vi "QAM_1.vi"() -> ()   [LabVIEW 2019]
uses:
  <vilib>/addons/Modulation/Analog/support/mod_Set Error Source.vi
  <vilib>/addons/Modulation/Digital/Support/Common/Validators/mod_AWGN Validate.vi
  <vilib>/addons/Modulation/Digital/Impairments/subVIs/mod_createSeeds.vi
  <vilib>/addons/Modulation/Digital/Support/Common/Validators/mod_Validate Samples Per Symbol.vi
  <vilib>/addons/Modulation/Analog/support/Validators/mod_Validate Complex Waveform.vi
  <vilib>/addons/Modulation/Analog/support/Validators/mod_WFErrorHandler.vi
  <vilib>/addons/Modulation/Digital/General/MT Generate QAM System Parameters(M).vi
  <vilib>/addons/Modulation/Digital/Support/Common/Validators/mod_Generate Filter Coefficients Validate.vi
  <vilib>/addons/Modulation/Digital/General/subVIs/mod_Generate Filter Coefficients.vi
  <vilib>/addons/Modulation/Digital/General/subVIs/mod_Generate Bits PN Sequence.vi
  <vilib>/Analysis/1siggen.llb/Gaussian White Noise (obs 90).vi
  <vilib>/addons/Modulation/Analog/MT Upconvert Baseband (Real).vi
  <vilib>/express/express analysis/Spectral/Block/exnSpectralBlock spectral measurements RMS poly.vi
  <vilib>/express/express analysis/Spectral/Block/exnSpectralBlock spectral measurements RMS DDT.vi
  <vilib>/express/express analysis/Spectral/XNode/ExpressSpectralMeasurementsBlockNode.xnode
  <vilib>/addons/Modulation/niDMT.lvlib
  <vilib>/addons/Modulation/niAMT.lvlib
panel:
  in  "pulse shaping filter (none)":T1(ring)
  in  "?":T2(tab)
  out "Upconverted Waveform":waveform(dbl)(graph)
  out "Constellation Graph":T3(graph)
  out "FFT (RMS)":dynamicdata(graph)
  out "Match Found?":bool
  in  "carrier frequency (Hz)":dbl min=-0.5 max=0.5 format="%.0p"
  in  "stop":bool
  in  "autoscale":bool
  in  "Eb/N0 (10 dB)":dbl=10.0 format="%.0p"
  out "Demodulated String":string
  in  "symbol rate (Hz)":dbl=1.0 format="%.0p"
  in  "Add Bit Padding":bool
  in  "Message to send":string
  in  "M-QAM (16)":u16(ring) items=["4"=4, "8"=8, "16"=16, "32"=32]
  in  "Reset":bool
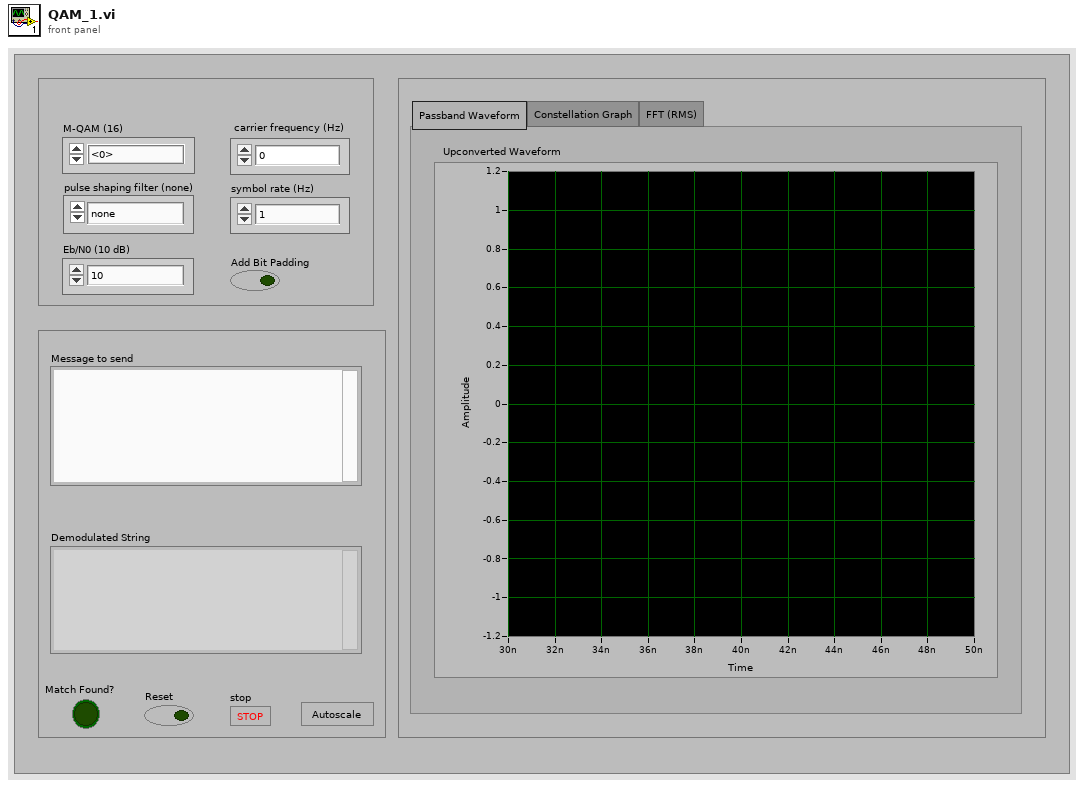
[diagram p1: front panel]
types:
  T1 = enum16{"none", "Raised Cosine", "Root Raised Cos", "Gaussian"}
  T2 = enum32{"Passband Waveform", "Constellation Graph", "FFT (RMS)"}
  T3 = cluster{"Decimated Array":dbl[], "Decimated Array":dbl[]}[]
  T4 = enum16{"FSK", "PSK", "QAM", "MSK", "PAM", "ASK", "CPM"}
  T5 = cluster{"averaging mode":u16, "weighting mode":u16, "number of averages":u32}
  T6 = cluster{"dB On (F)":bool, "unwrap phase (F)":bool, "convert to degree (F)":bool}
  T7 = cluster{"samples per symbol (16)":i32, "symbol map":cdb[]}
  T8 = typedef "niAMT.lvlib/Complex Data Waveform.ctl" = cluster{"t0":dbl, "dt":dbl, "Y":cdb[]}
  T9 = cluster{"constellation":dbl[], "oversampled data":dbl[]}[]
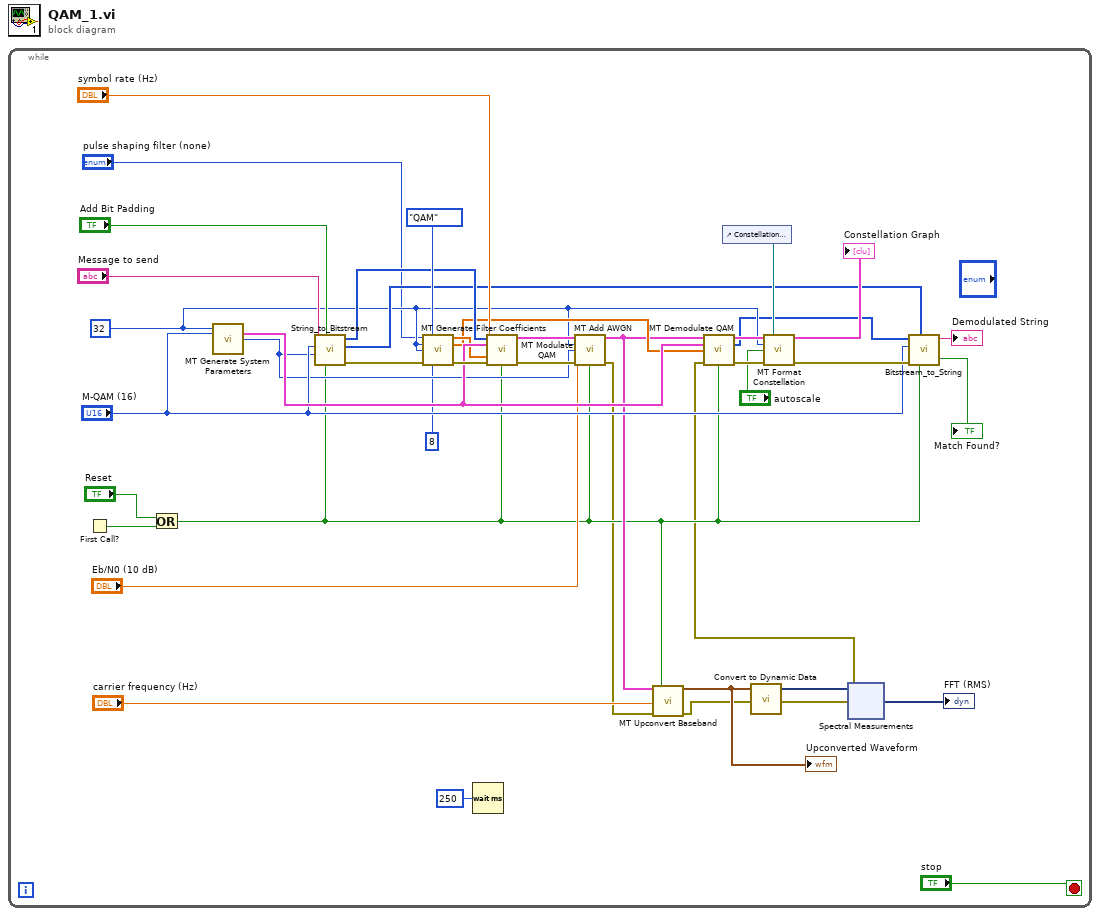
[diagram p0: block diagram]
diagram:
  n1 = while {
    stop <- "stop" stop-if-true
    w13 = 32 ("samples per symbol (16)")
    n2 = First Call?() -> (First Call?: T/F=w38:bool)
    n3 = Or(x="Reset", y=w38) -> (x .or. y?=w5:bool)
    n4 = call-poly <vilib>:"MT Generate System Parameters.vi"("samples per symbol (16)"=w13, "M-QAM (16)"="M-QAM (16)") -> ("QAM system parameters"=w23:T7, "bits per symbol"=w20:i32)  [unwired: 11 in, 1 out]
    n5 = call "String_to_Bitstream.vi"("Reset"=w5, "Add Bit Padding"="Add Bit Padding", "Guard Bits to Add"=w20, "M-ary (16)"="M-QAM (16)", "InputStrig"="Message to send") -> ("error out"=w31:errorcluster, "Character Array"=w32:u8[], "Bitstream (with Guard Bits)"=w33:i8[])  [unwired: 1 in, 2 out]
    n6 = call <vilib>:"MT Generate Filter Coefficients.vi"("pulse shaping filter (none)"="pulse shaping filter (none)", "modulation type"=T4."QAM", "pulse shaping samples per symbol (16)"=w13, "matched samples per symbol (16)"=w13, "error in (no error)"=w31, "filter length (symbols)"=8) -> ("pulse shaping filter coefficients"=w19:dbl[], "matched filter coefficients"=w18:dbl[], "error out"=w30:errorcluster)  [unwired: 7 in]
    n7 = Wait (ms)(milliseconds to wait=u32 250) -> ()  [unwired: 1 out]
    n8 = call <vilib>:"MT Modulate QAM.vi"("input bit stream"=w33, "QAM system parameters"=w23, "symbol rate (Hz)"="symbol rate (Hz)", "pulse shaping filter coefficients"=w19, "error in (no error)"=w30, "reset? (T)"=w5) -> ("output complex waveform"=w24:T8, "error out"=w29:errorcluster)  [unwired: 7 in, 1 out]
    n9 = call <vilib>:"MT Add AWGN.vi"("input complex waveform"=w24, "samples per symbol (16)"=w13, "bits per symbol (1)"=w20, "Eb/N0 (10 dB)"="Eb/N0 (10 dB)", "error in (no error)"=w29, "reset? (T)"=w5) -> ("output complex waveform"=w7:T8, "error out"=w4:errorcluster)  [unwired: 7 in, 1 out]
    n10 = call-poly <vilib>:"MT Upconvert Baseband.vi"("baseband waveform (complex)"=w7, "reset? (F)"=w5, "carrier frequency (Hz)"="carrier frequency (Hz)", "error in (no error)"=w4) -> ("passband waveform"=w16:waveform(dbl), "error out"=w3:errorcluster)  [unwired: 10 in]
    "Upconverted Waveform" <- w16
    n11 = control-ref of="Constellation Graph"() -> (w41:refnum<vi>)
    n12 = call "Convert to Dynamic Data"("Waveform"=w16) -> ("Dynamic Data Type"=w17:dynamicdata)  [unwired: 3 in]
    n13 = xnode "Spectral Measurements"("Signals"=w17, "error in (no error)"=w3) -> ("Measurement Output"=→"FFT (RMS)":dynamicdata, "error out"=w2:errorcluster)  [unwired: 1 out]
    n14 = call <vilib>:"MT Demodulate QAM.vi"("input complex waveform"=w7, "QAM system parameters"=w23, "matched filter coefficients"=w18, "error in (no error)"=w2, "reset? (T)"=w5) -> ("recovered complex waveform"=w25:T8, "output bit stream"=w12:i8[], "error out"=w28:errorcluster)  [unwired: 6 in, 2 out]
    n15 = call <vilib>:"MT Format Constellation.vi"("waveform"=w25, "constellation reference"=w41, "samples per symbol"=w13, "autoscale"="autoscale", "error in (no error)"=w28) -> ("constellation graph"=→"Constellation Graph":T9, "error out"=w27:errorcluster)  [unwired: 9 out]
    n16 = call "Bitstream_to_String.vi"("Reset"=w5, "Character Array"=w32, "error in (no error)"=w27, "M-ary (16)"="M-QAM (16)", "Bit Array"=w12) -> ("Demodulated String"=→"Demodulated String":string, "Match Found?"=→"Match Found?":bool)  [unwired: 1 in, 4 out]
  }
